vi "Jenkins Unit Test_2.vi"(11 "Args":string[](array[string])) -> (2 "Output":string, 3 "Exit Code":i32)   [LabVIEW 2021]
uses:
  <vilib>/addons/_JKI Toolkits/Caraya/classes/Test Suite/Define Test Suite (JUnit Report).vi
  <vilib>/addons/_JKI Toolkits/Caraya/classes/Test Suite/Test Suite.lvclass
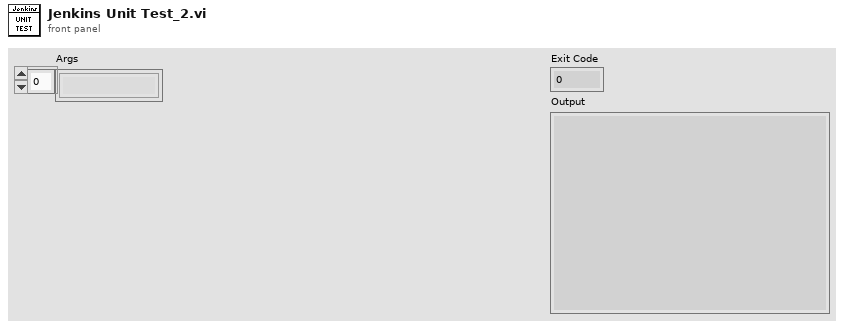
[diagram p1: front panel]
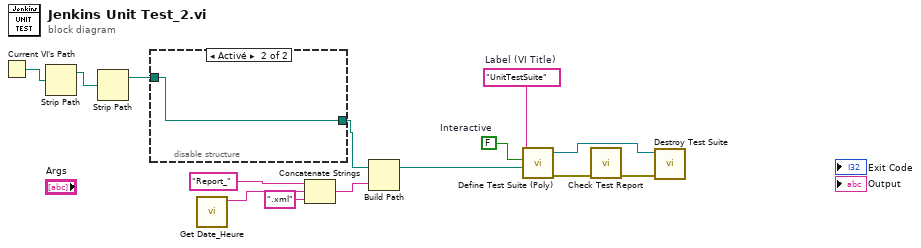
[diagram p0: block diagram]
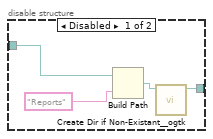
[diagram p2: hidden frame]
diagram:
  w13 = FALSE  # Interactive
  w14 = "UnitTestSuite"  # Label (VI Title)
  n1 = Current VI's Path() -> (path=w5:path)
  n2 = Strip Path(path=w5) -> (stripped path=w4:path)  [unwired: 1 out]
  n3 = Strip Path(path=w4) -> (stripped path=w3:path)  [unwired: 1 out]
  n4 = disable-structure shown="Activé" {
    disable-tunnel: [w16 w19] -> w10
    disable-tunnel: w3 -> [w15 w19]
    frame Disabled {
      n5 = Build Path(base path=w15, name or relative path="Reports") -> (appended path=w17:path)
      n6 = call <userlib>:"Create Dir if Non-Existant__ogtk.vi"("Directory Path"=w17) -> ("dup Directory Path"=w16:path)  [unwired: 8 in, 2 out]
    }
    frame Enabled {
    }
  }
  n7 = call "Get Date_Heure.vi"() -> ("Date_Heure"=w7:string)  [unwired: 11 in]
  n8 = Concatenate Strings("Report_" ("Report Path"), w7, ".xml" ("chaîne")) -> (w9:string)
  n9 = Build Path(base path=w10, name or relative path=w9) -> (appended path=w12:path)
  n10 = call-poly <vilib>:"Define Test Suite (Poly).vi"("Report Path"=w12, "Interactive"=w13, "Label (VI Title)"=w14) -> ("error out"=w2:errorcluster, "Test Suite"=w6:refnum<class "Test Suite.lvclass">)  [unwired: 6 in, 1 out]
  n11 = call "Check Test Report.vi"("error in (no error)"=w2) -> ("error out"=w1:errorcluster)  [unwired: 10 in]
  n12 = call-dynamic "Destroy Test Suite.vi"("error in (no error)"=w1, "Test Suite in"=w6) -> ()  [unwired: 8 in, 2 out]
